vi "Read Request Queue.vi"(8 "error in (no error)":errorcluster, 11 "Abstract Init Parameters in":refnum<class "Abstract Init Parameters.lvclass">) -> (0 "error out":errorcluster, 2 "Message Queue Library.lvlib:Abstract Message Queue.lvclass":refnum<class "Abstract Message Queue.lvclass">, 3 "Abstract Init Parameters out":refnum<class "Abstract Init Parameters.lvclass">)   [LabVIEW 2017, in "Messaging.lvlib" / "Abstract Init Parameters.lvclass"]
uses:
  Abstract Init Parameters.lvclass
  Message Queue/Abstract Message Queue/Abstract Message Queue.lvclass
  Abstract Init Parameters.lvclass/Abstract Init Parameters.ctl
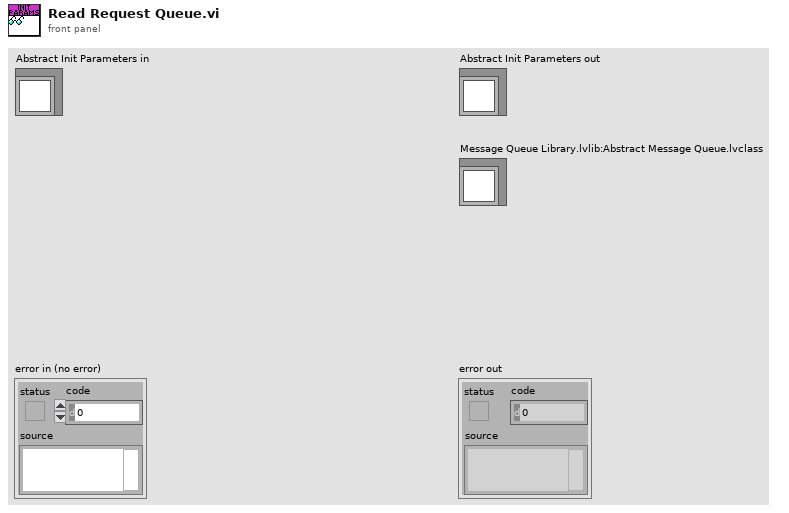
[diagram p1: front panel]
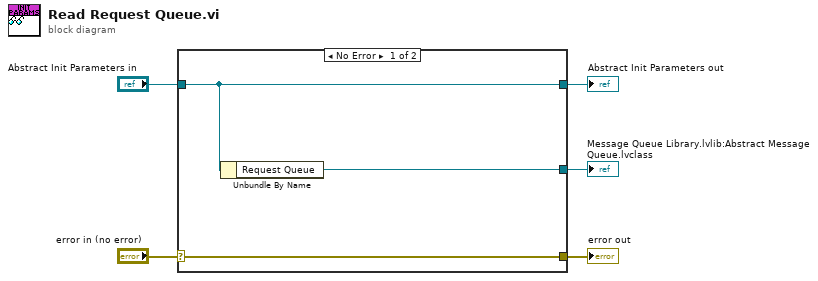
[diagram p0: block diagram]
diagram:
  n1 = case shown="No Error" "error in (no error)" {
    selector: "error in (no error)" -> [w8 w9]
    tunnel: [w8 w9] -> w4
    tunnel: [w7 w10] -> w2
    tunnel: "Abstract Init Parameters in" -> [w7 w10]
    tunnel: [w6 _] -> w1
    frame No Error {
      n2 = Unbundle By Name(w7) -> ("Request Queue"=w6:refnum<class "Abstract Message Queue.lvclass">)
    }
    frame Error {
    }
  }
  "error out" <- w4
  "Abstract Init Parameters out" <- w2
  "Message Queue Library.lvlib:Abstract Message Queue.lvclass" <- w1
